vi "sub_vi_noise.vi"(0 "x1":dbl, 2 "y1":dbl, 3 "x2":dbl, 4 "sigma":dbl[](array[numeric]), 5 "y2":dbl) -> (7 "Noise":dbl[](array[numeric]))   [LabVIEW 2016]
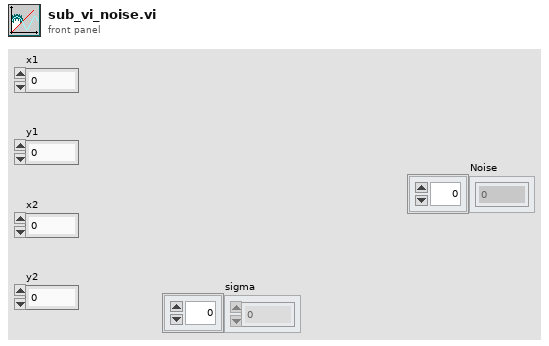
[diagram p1: front panel]
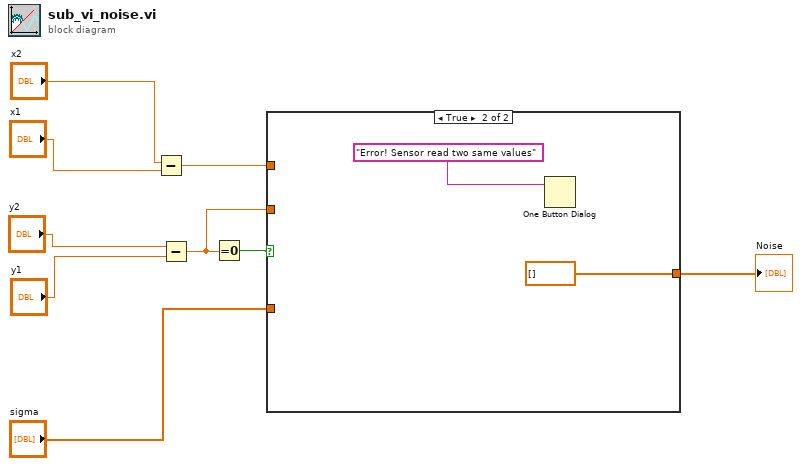
[diagram p0: block diagram]
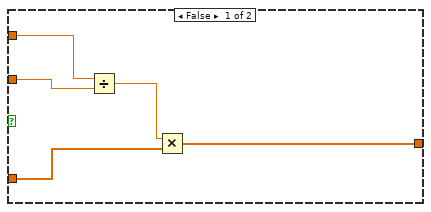
[diagram p2: hidden frame]
diagram:
  n1 = Subtract(x="x2", y="x1") -> (x-y=w4:dbl)
  n2 = Subtract(x="y2", y="y1") -> (x-y=w2:dbl)
  n3 = Equal To 0?(x=w2) -> (x = 0?=w5:bool)
  n4 = case shown="True" w5 {
    tunnel: w4 -> [w14 _]
    tunnel: "sigma" -> [w11 _]
    tunnel: [w10 dbl[] []] -> w1
    tunnel: w2 -> [w13 _]
    frame False {
      n5 = Divide(x=w14, y=w13) -> (x/y=w12:dbl)
      n6 = Multiply(x=w12, y=w11) -> (x*y=w10:dbl[])
    }
    frame True {
      n7 = One Button Dialog(message="Error! Sensor read two same values") -> ()  [unwired: 1 in, 1 out]
    }
  }
  "Noise" <- w1
